vi "Paw-Control_Api.vi"(6 "I2C Ref In":T1={"myRIO Reference"={"myRIO Model"=enum."Unknown", "myRIO Hardware Reference"={"Generic FPGA Reference"=refnum, "Allow multiple opens"=FALSE}}, "I2C Channels Enum"=enum."Not Connected", "I2C Configuration"={"I2C Transfer Rate"=enum."Fast mode (400 kbps)"}}, 8 "Error In":errorcluster, 11 "夾爪動作":enum16{"開", "合"}(ring)) -> (0 "error out":errorcluster)   [LabVIEW 2019]
uses:
  <vilib>/myRIO/Instrument Drivers/Onboard IO/I2C/typedefs/I2C Reference.ctl
  <vilib>/myRIO/Common/Instrument Driver Framework/Utilities/typedefs/myRIO Generic Hardware Reference.ctl
  <vilib>/myRIO/Common/Instrument Driver Framework/Utilities/typedefs/Hardware Version Enum.ctl
  <vilib>/myRIO/Common/Instrument Driver Framework/Utilities/typedefs/myRIO v1.0 Reference.ctl
  <vilib>/myRIO/Common/Instrument Driver Framework/Utilities/typedefs/Generic FPGA Reference.ctl
  <vilib>/myRIO/Common/Instrument Driver Framework/myRIO v1.0/I2C/typedefs/I2C Channels Enum.ctl
  <vilib>/myRIO/Instrument Drivers/Onboard IO/I2C/typedefs/I2C Configuration.ctl
  <vilib>/myRIO/Instrument Drivers/Onboard IO/I2C/typedefs/I2C Transfer Rate.ctl
  <vilib>/myRIO/Instrument Drivers/Onboard IO/I2C/I2C.lvlib
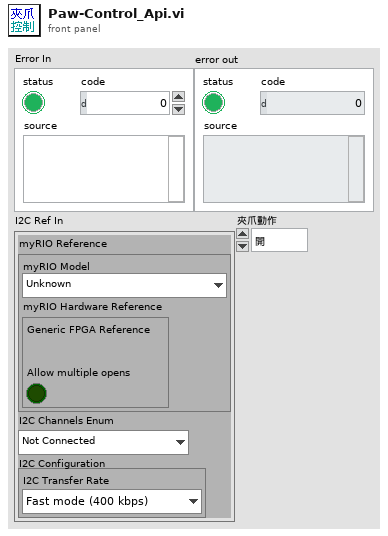
[diagram p1: front panel]
types:
  T1 = typedef "I2C.lvlib/I2C Reference.ctl" = cluster{"myRIO Reference":T2, "I2C Channels Enum":T6, "I2C Configuration":T7}
  T2 = typedef "myRIO Generic Hardware Reference.ctl" = cluster{"myRIO Model":T3, "myRIO Hardware Reference":T4}
  T3 = typedef "Hardware Version Enum.ctl" = enum16{"Unknown", "myRIO-1900", "myRIO-1950", "roboRIO", "NI ELVIS RIO CM", "ELVIS III"}
  T4 = typedef "myRIO v1.0 Reference.ctl" = cluster{"Generic FPGA Reference":T5, "Allow multiple opens":bool}
  T5 = typedef "Generic FPGA Reference.ctl" = refnum<k20>
  T6 = typedef "I2C Channels Enum.ctl" = enum16{"Not Connected", "A/I2C", "B/I2C", "I2C/I2C"}
  T7 = typedef "I2C.lvlib/I2C Configuration.ctl" = cluster{"I2C Transfer Rate":T8}
  T8 = typedef "I2C.lvlib/I2C Transfer Rate.ctl" = enum16{"Standard mode (100 kbps)", "Fast mode (400 kbps)"}
  T9 = enum16{"LED/PWM00", "LED/PWM01", "LED/PWM02", "LED/PWM03", "LED/PWM04", "LED/PWM05", "LED/PWM06", "LED/PWM07", "LED/PWM08", "LED/PWM09", "LED/PWM10", "LED/PWM11", "LED/PWM12", "LED/PWM13", "LED/PWM14", "LED/PWM15"}
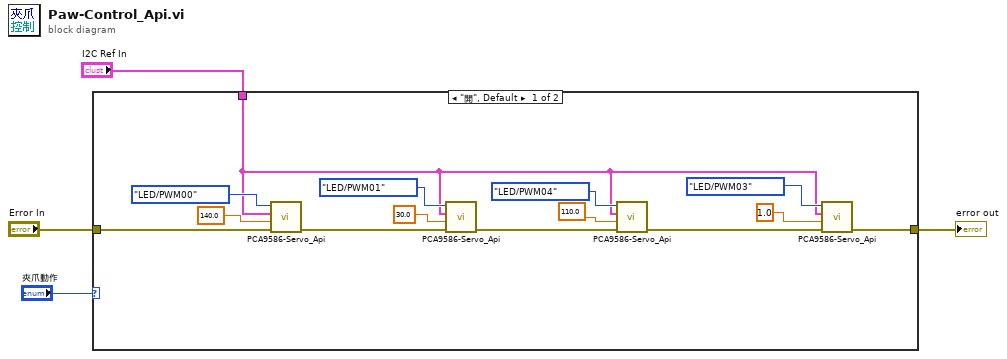
[diagram p0: block diagram]
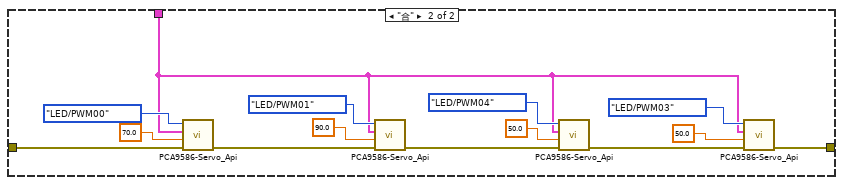
[diagram p2: hidden frame]
diagram:
  n1 = case shown="\"開\", Default" "夾爪動作" {
    tunnel: [w6 w20] -> w4
    tunnel: "Error In" -> [w10 w24]
    tunnel: "I2C Ref In" -> [w5 w19]
    frame "開", Default {
      n2 = call "PCA9586-Servo_Api.vi"("Error In"=w10, "角度"=140.0, "I2C Ref In"=w5, "PWM腳位"=T9."LED/PWM00") -> ("Error Out"=w9:errorcluster)  [unwired: 7 in]
      n3 = call "PCA9586-Servo_Api.vi"("Error In"=w9, "角度"=30.0, "I2C Ref In"=w5, "PWM腳位"=T9."LED/PWM01") -> ("Error Out"=w8:errorcluster)  [unwired: 7 in]
      n4 = call "PCA9586-Servo_Api.vi"("Error In"=w8, "角度"=110.0, "I2C Ref In"=w5, "PWM腳位"=T9."LED/PWM04") -> ("Error Out"=w7:errorcluster)  [unwired: 7 in]
      n5 = call "PCA9586-Servo_Api.vi"("Error In"=w7, "角度"=1.0, "I2C Ref In"=w5, "PWM腳位"=T9."LED/PWM03") -> ("Error Out"=w6:errorcluster)  [unwired: 7 in]
    }
    frame "合" {
      n6 = call "PCA9586-Servo_Api.vi"("Error In"=w24, "角度"=70.0, "I2C Ref In"=w19, "PWM腳位"=T9."LED/PWM00") -> ("Error Out"=w23:errorcluster)  [unwired: 7 in]
      n7 = call "PCA9586-Servo_Api.vi"("Error In"=w23, "角度"=90.0, "I2C Ref In"=w19, "PWM腳位"=T9."LED/PWM01") -> ("Error Out"=w22:errorcluster)  [unwired: 7 in]
      n8 = call "PCA9586-Servo_Api.vi"("Error In"=w22, "角度"=50.0, "I2C Ref In"=w19, "PWM腳位"=T9."LED/PWM04") -> ("Error Out"=w21:errorcluster)  [unwired: 7 in]
      n9 = call "PCA9586-Servo_Api.vi"("Error In"=w21, "角度"=50.0, "I2C Ref In"=w19, "PWM腳位"=T9."LED/PWM03") -> ("Error Out"=w20:errorcluster)  [unwired: 7 in]
    }
  }
  "error out" <- w4
